vi "Tester.vi"() -> ()   [LabVIEW 2016]
uses:
  <vilib>/Analysis/1siggen.llb/Ramp Pattern by Samples.vi
  <vilib>/Analysis/2dsp.llb/Decimate (single shot, DBL).vi
  <vilib>/Analysis/NI_AALBase.lvlib
  <vilib>/Analysis/NI_AALPro.lvlib
  Waveform Equalizer/Waveform Equalizer.lvlib
panel:
  out "Waveform Graph":waveform(dbl)[](graph)
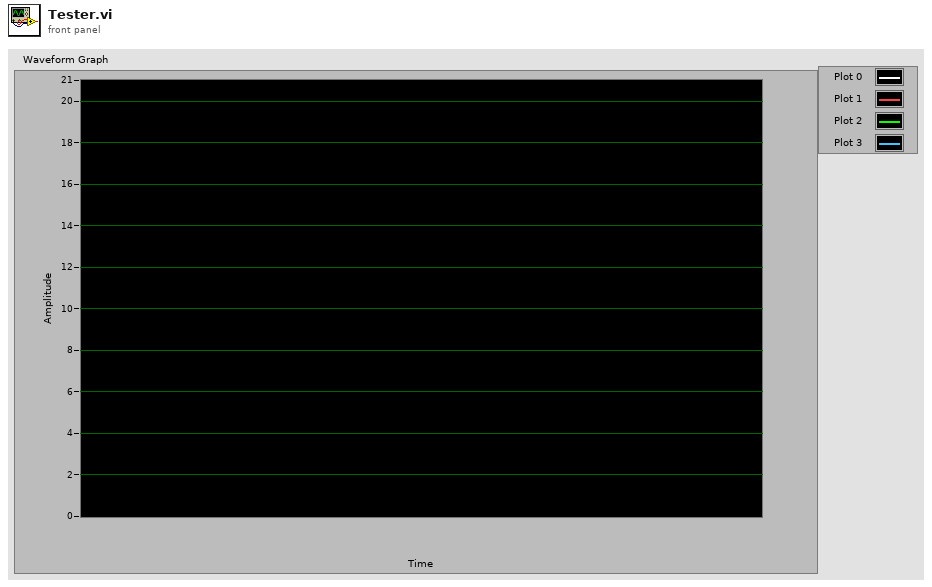
[diagram p1: front panel]
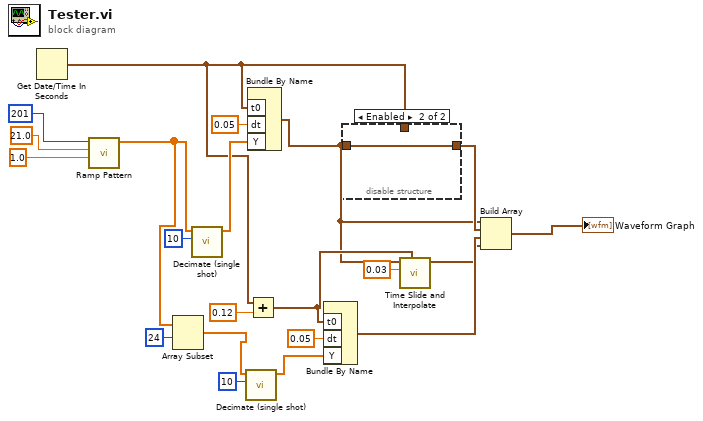
[diagram p0: block diagram]
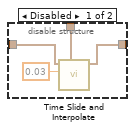
[diagram p2: hidden frame]
diagram:
  n1 = Get Date/Time In Seconds() -> (seconds since 1Jan1904=w11:timestamp)
  n2 = call-poly <vilib>:"Ramp Pattern.vi"("start"=1.0, "end"=21.0, "samples"=201) -> ("Ramp Pattern"=w13:dbl[])  [unwired: 7 in, 1 out]
  n3 = Array Subset(array=w13, index=24) -> (w7:dbl[])  [unwired: 1 in]
  n4 = call-poly <vilib>:"Decimate (single shot).vi"("decimating factor"=10, "X"=w13) -> ("Decimated Array"=w15:dbl[])  [unwired: 8 in, 1 out]
  n5 = call-poly <vilib>:"Decimate (single shot).vi"("decimating factor"=10, "X"=w7) -> ("Decimated Array"=w6:dbl[])  [unwired: 8 in, 1 out]
  n6 = Bundle By Name("t0"=w11, "dt"=0.05, "Y"=w15) -> (w1:waveform(dbl))  [unwired: 1 in]
  n7 = Add(x=w11, y=0.12) -> (x+y=w4:timestamp)
  n8 = Bundle By Name("t0"=w4, "dt"=0.05, "Y"=w6) -> (w8:waveform(dbl))  [unwired: 1 in]
  n9 = disable-structure shown="Enabled" {
    disable-tunnel: [w25 w26] -> w14
    disable-tunnel: w11 -> [w23 _]
    disable-tunnel: w1 -> [w22 w26]
    frame Disabled {
      n10 = call "Time Slide and Interpolate.vi"("Target t0"=w23, "Target dt"=0.03, "input waveform"=w22) -> ("output waveform"=w25:waveform(dbl))  [unwired: 8 in]
    }
    frame Enabled {
    }
  }
  n11 = call "Time Slide and Interpolate.vi"("Target t0"=w4, "Target dt"=0.03, "input waveform"=w1) -> ("output waveform"=w2:waveform(dbl))  [unwired: 8 in]
  n12 = Build Array(w1, w14, w8, w2) -> (→"Waveform Graph":waveform(dbl)[])
